vi "PRN Generation_Station1.vi"(0 "Part PRN QR":path, 3 "error in (no error)":errorcluster, 4 "Cluster":T2) -> (6 "QR Code":string, 7 "PRN to Print":string, 10 "error out":errorcluster)   [LabVIEW 2017]
uses:
  Controls/Recipe.ctl
  <vilib>/addons/database/Connection.llb/Conn ObjectReference.ctl
  <vilib>/addons/database/NI_Database_API.lvlib
panel:
  in  "Ref Data":T3={"Ass. Sensor Select"={"Ass. Sensor Select"=FALSE, "Camera-1 \nProg No."=0, "Camera-2 \nProg No."=0, "Gun \nProg No."=0}, "Torque Sensor Select"={"Torque Sensor-1"=FALSE, "Torque Sensor-2"=FALSE, "Torque Sensor-3"=FALSE, "Torque Sensor-4"=FALSE, "Torque Sensor-5"=FALSE, "Torque Sensor-6"=FALSE, "Torque Sensor-7"=FALSE, "Torque Sensor-8"=FALSE, "Torque Sensor-9"=FALSE, "Torque Sensor-10"=FALSE, "Torque Sensor-11"=FALSE, "Torque Sensor-12"=FALSE}, "Bin Seq. Select"={"First Bin"=0, "Second Bin"=0, "Third Bin"=0, "Fourth Bin"=0, "Fifth Bin"=0, "Sixth Bin"=0, "Seventh Bin"=0, "Eighth Bin"=0, "Camera-1 Trig"=0, "Camera-2 Trig"=0}, "T-Bin Seq. Select"={"First"=0, "Second"=0, "Third"=0, "Fourth"=0, "Fifth"=0, "Sixth"=0}, "Reference Barcode"={"Spring Barcode"="", "Body Barcode"="", "14 Char of Barcode"="", "Final Barcode Length"="26"}, "Label Data"={"Cust. Part No."="", "TML Part No."="", "Vendor Code"="", "Revision Level"="", "Part Description"="", "Vendor Name"=""}} {"T-Bin Seq. Select"."First" max=8 step=1; "T-Bin Seq. Select"."Second" max=8 step=1; "T-Bin Seq. Select"."Third" max=8 step=1; "T-Bin Seq. Select"."Fourth" max=8 step=1; "T-Bin Seq. Select"."Fifth" max=8 step=1; "T-Bin Seq. Select"."Sixth" max=8; "Ass. Sensor Select"."Gun \nProg No." max=8 step=1; "Ass. Sensor Select"."Camera-2 \nProg No." max=8 step=1; "Ass. Sensor Select"."Camera-1 \nProg No." max=8 step=1}
  # "Bin No."
  # "Bin No."
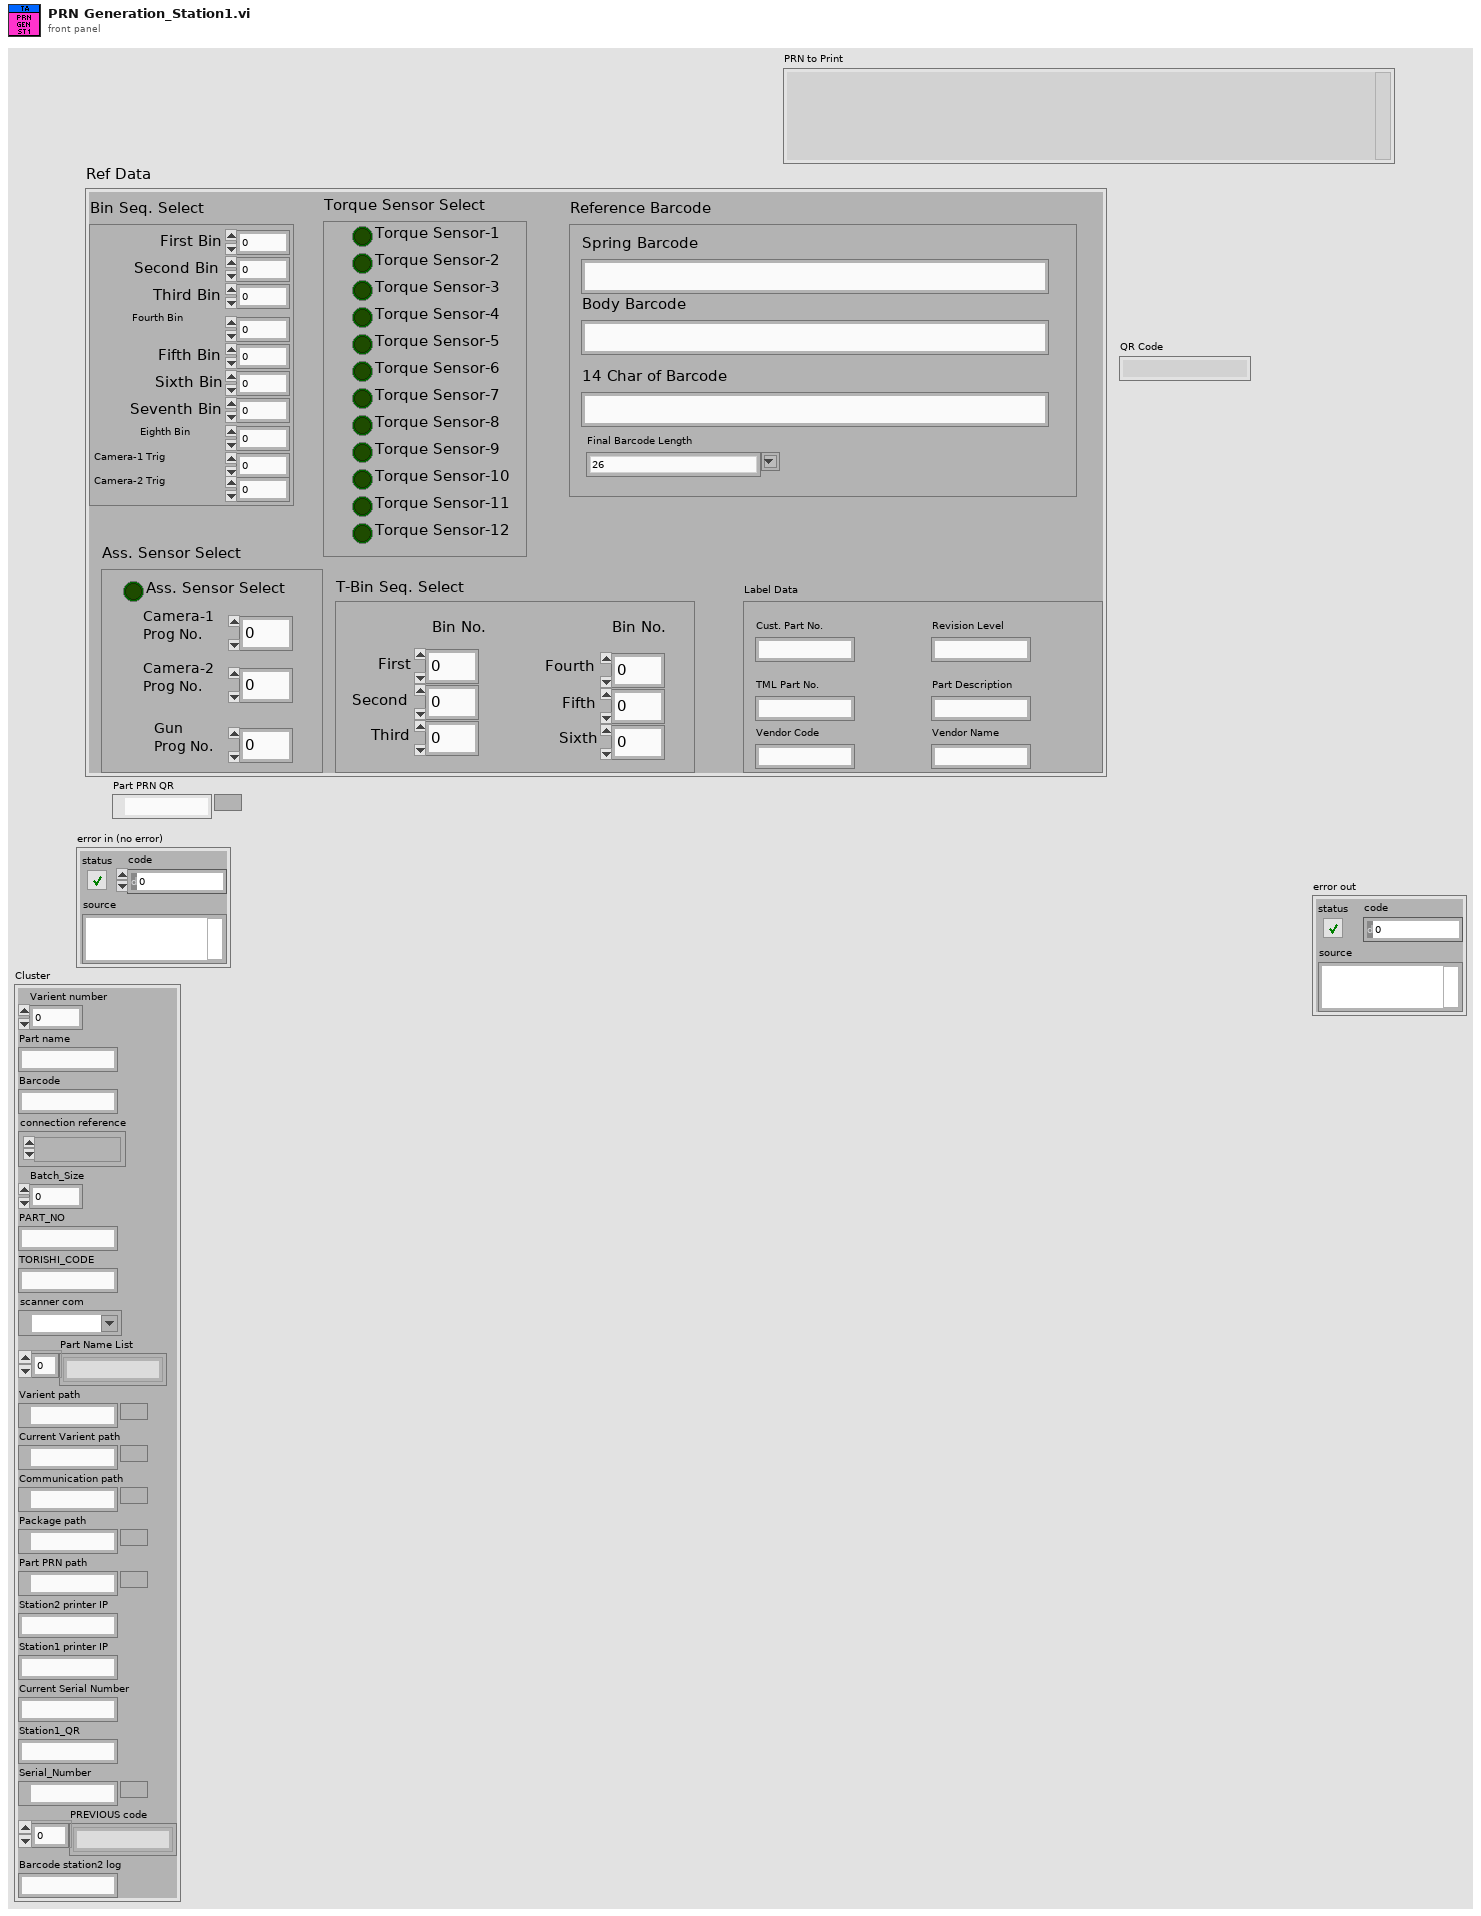
[diagram p1: front panel]
types:
  T1 = typedef "NI_Database_API.lvlib/Conn ObjectReference.ctl" = refnum<k1>
  T2 = cluster{"Varient number":u16, "Part name":string, "Barcode":string, "connection reference":T1, "Batch_Size":u16, "PART_NO":string, "TORISHI_CODE":string, "scanner com":refnum<visa-resource-name>, "Part Name List":string[], "Varient path":path, "Current Varient path":path, "Communication path":path, "Package path":path, "Part PRN path":path, "Station2 printer IP":string, "Station1 printer IP":string, "Current Serial Number":string, "Station1_QR":string, "Serial_Number":path, "PREVIOUS code":string[], "Barcode station2 log":string}
  T3 = typedef "Recipe.ctl" = cluster{"Ass. Sensor Select":cluster{"Ass. Sensor Select":bool, "Camera-1 \nProg No.":u16, "Camera-2 \nProg No.":u16, "Gun \nProg No.":u16}, "Torque Sensor Select":cluster{"Torque Sensor-1":bool, "Torque Sensor-2":bool, "Torque Sensor-3":bool, "Torque Sensor-4":bool, "Torque Sensor-5":bool, "Torque Sensor-6":bool, "Torque Sensor-7":bool, "Torque Sensor-8":bool, "Torque Sensor-9":bool, "Torque Sensor-10":bool, "Torque Sensor-11":bool, "Torque Sensor-12":bool}, "Bin Seq. Select":cluster{"First Bin":u16, "Second Bin":u16, "Third Bin":u16, "Fourth Bin":u16, "Fifth Bin":u16, "Sixth Bin":u16, "Seventh Bin":u16, "Eighth Bin":u16, "Camera-1 Trig":u16, "Camera-2 Trig":u16}, "T-Bin Seq. Select":cluster{"First":u16, "Second":u16, "Third":u16, "Fourth":u16, "Fifth":u16, "Sixth":u16}, "Reference Barcode":cluster{"Spring Barcode":string, "Body Barcode":string, "14 Char of Barcode":string, "Final Barcode Length":string}, "Label Data":cluster{"Cust. Part No.":string, "TML Part No.":string, "Vendor Code":string, "Revision Level":string, "Part Description":string, "Vendor Name":string}}
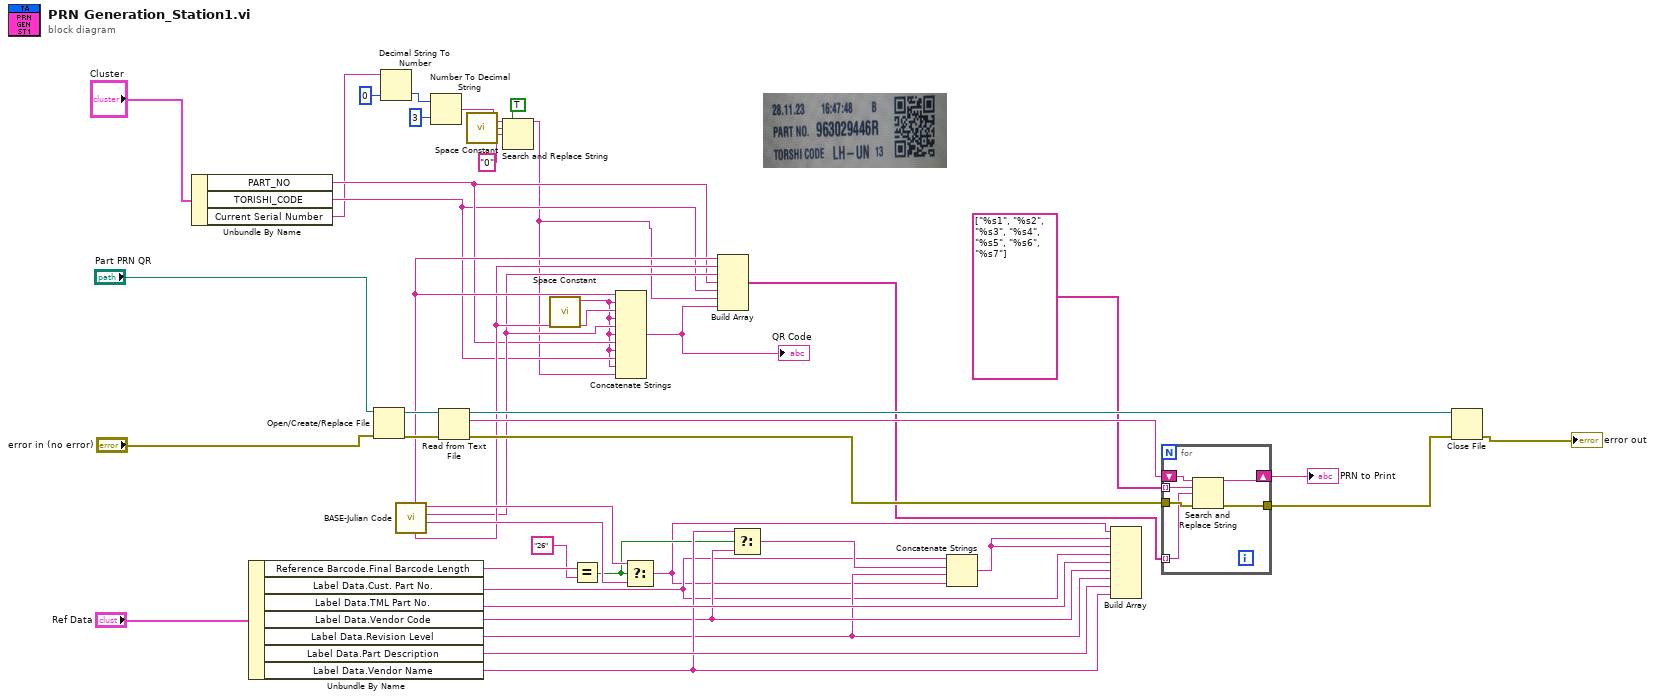
[diagram p0: block diagram]
diagram:
  n1 = Unbundle By Name("Cluster") -> ("PART_NO"=w14:string, "TORISHI_CODE"=w13:string, "Current Serial Number"=w2:string)
  n2 = Unbundle By Name("Ref Data") -> ("Reference Barcode.Final Barcode Length"=w32:string, "Label Data.Cust. Part No."=w21:string, "Label Data.TML Part No."=w28:string, "Label Data.Vendor Code"=w25:string, "Label Data.Revision Level"=w23:string, "Label Data.Part Description"=w27:string, "Label Data.Vendor Name"=w26:string)
  n3 = Open/Create/Replace File(file path (use dialog)="Part PRN QR", error in="error in (no error)") -> (refnum out=w41:refnum<file>, error out=w42:errorcluster)  [unwired: 4 in, 1 out]
  n4 = Decimal String To Number(string=w2, default (0L)=0 ("default (0 I32)")) -> (number=w8:i32)  [unwired: 1 in, 1 out]
  n5 = call "BASE-Julian Code.vi"() -> ("Short Date"=w29:string, "Shift"=w15:string, "Julian Code"=w30:string, "Long time with :"=w16:string, "Long date with /"=w17:string)  [unwired: 6 in, 1 out]
  n6 = Number To Decimal String(number=w8, width (-)=i16 3) -> (decimal integer string=w6:string)
  n7 = Read from Text File(file (use dialog)=w41, error in=w42) -> (refnum out=w43:refnum<file>, text=w39:string, error out=w37:errorcluster)  [unwired: 2 in, 1 out]
  n8 = call <vilib>:"Space Constant.vi"() -> ("String"=w5:string)
  n9 = Search and Replace String(replace all?=TRUE ("replace all? (F)"), input string=w6, search string=w5, replace string="0" ("replace string (\"\")")) -> (result string=w1:string)  [unwired: 4 in, 3 out]
  n10 = call <vilib>:"Space Constant.vi"() -> ("String"=w12:string)
  n11 = Equal?(x=w32, y="26") -> (x = y?=w22:bool)
  n12 = Concatenate Strings(w17, w12, w16, w12, w15, w12, w14, w12, w13, w12, w1) -> (w10:string)
  "QR Code" <- w10
  n13 = Select(t=w30, s=w22, f=w29) -> (s? t:f=w20:string)
  n14 = Build Array(w17, w16, w15, w14, w13, w1, w10) -> (w11:string[])
  n15 = Select(t=w26, s=w22, f=w25) -> (s? t:f=w24:string)
  n16 = Concatenate Strings(w21, w24, w23, w20) -> (w34:string)
  n17 = Build Array(w20, w34, w34, w21, w28, w25, w23, w27, w26) -> ()  [unwired: 1 out]
  n18 = for {
    shift-right: [w49] -> w38
    shift-left: w39 -> [w50]
    tunnel: w37 -> [w48]
    tunnel: [w47] -> w36
    tunnel: string[] ["%s1", "%s2", "%s3", "%s4", "%s5", "%s6", "%s7"] -> [w46] mode=indexing
    tunnel: w11 -> [w45] mode=indexing
    n19 = Search and Replace String(input string=w50, search string=w46, replace string=w45, error in=w48) -> (result string=w49:string, error out=w47:errorcluster)  [unwired: 4 in, 2 out]
  }
  "PRN to Print" <- w38
  n20 = Close File(refnum=w43, error in=w36) -> (error out=→"error out":errorcluster)  [unwired: 1 out]
